vi "WLAN Rx Test Fetch Results.vi"(8 "error in (no error)":errorcluster, 11 "Template Rx Test in":refnum<class "niDTS WLAN Rx Test.lvclass">) -> (0 "error out":errorcluster, 2 "Results":T1, 3 "Template Rx Test out":refnum<class "niDTS WLAN Rx Test.lvclass">)   [LabVIEW 2015, in "niDTS WLAN.lvlib" / "niDTS WLAN Rx Test.lvclass"]
uses:
  niDTS WLAN Rx Test.lvclass
  Includes/niDTS WLAN Rx Test INC Results.ctl
  niDTS WLAN Rx Test.lvclass/niDTS WLAN Rx Test.ctl
  niDTS WLAN.lvlib
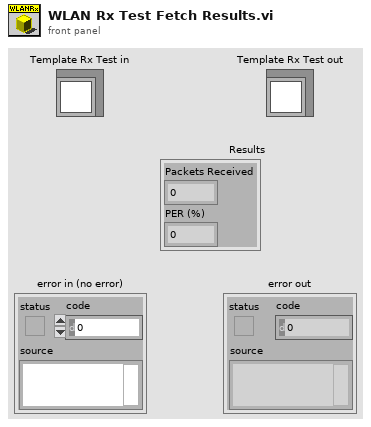
[diagram p1: front panel]
types:
  T1 = typedef "niDTS WLAN.lvlib/niDTS WLAN Rx Test INC Results.ctl" = cluster{"Packets Received":i32, "PER (%)":dbl}
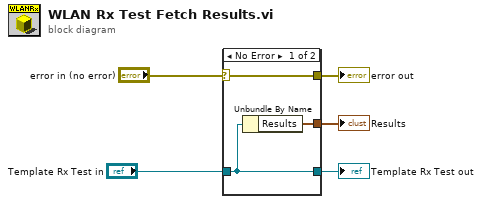
[diagram p0: block diagram]
diagram:
  n1 = case shown="No Error" "error in (no error)" {
    selector: "error in (no error)" -> [w6 w10]
    tunnel: [w6 w10] -> w4
    tunnel: [w8 w9] -> w2
    tunnel: "Template Rx Test in" -> [w8 w9]
    tunnel: [w7 _] -> w1
    frame No Error {
      n2 = Unbundle By Name(w8) -> ("Results"=w7:cluster{"Packets Received":i32, "PER":dbl})
    }
    frame Error {
    }
  }
  "error out" <- w4
  "Template Rx Test out" <- w2
  "Results" <- w1
